vi "AB_Engine_RTDEP_ProjURL_To_NetworkURL.vi"(8 "error in (no error)":errorcluster, 10 "libray ref":refnum<vi>, 11 "Project Refnum":refnum<vi>) -> (0 "error out":errorcluster)   [LabVIEW 2020]
uses:
  <vilib>/variable/NI_Variable.lvlib
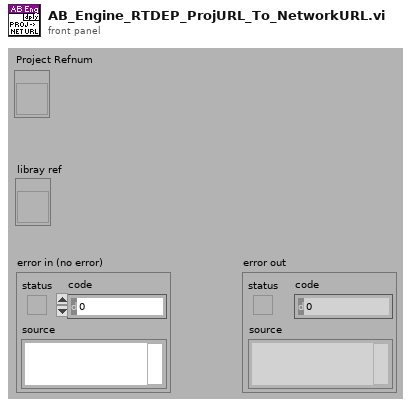
[diagram p1: front panel]
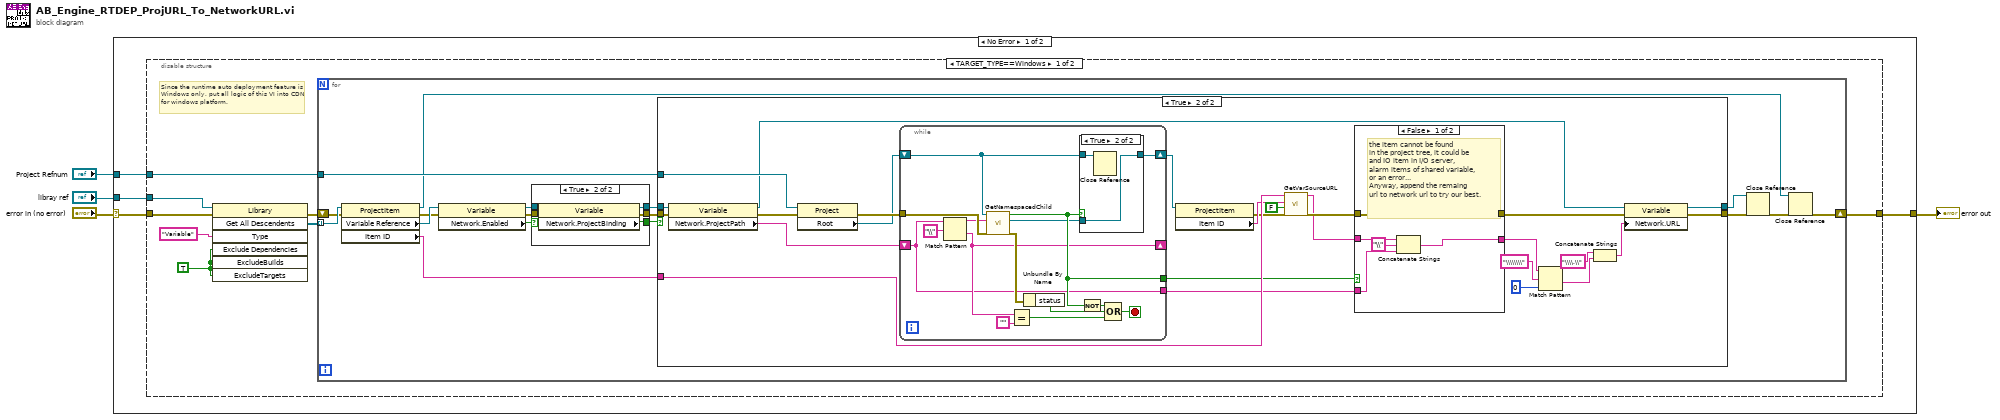
[diagram p0: block diagram]
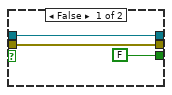
[diagram p2: hidden frame]
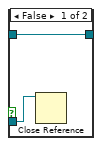
[diagram p5: hidden frame]
diagram:
  n1 = case shown="No Error" "error in (no error)" {
    selector: "error in (no error)" -> [w5 w97]
    tunnel: "Project Refnum" -> [w8 _]
    tunnel: [w7 w97] -> w3
    tunnel: "libray ref" -> [w6 _]
    frame No Error {
      n2 = disable-structure shown="TARGET_TYPE==Windows" {
        disable-tunnel: w8 -> [w16 _]
        disable-tunnel: [w11 w96] -> w7
        disable-tunnel: w6 -> [w10 _]
        disable-tunnel: w5 -> [w9 w96]
        frame condition #0 (active) {
          w14 = TRUE
          # "Since the runtime auto deployment feature is Windows only, put all logic of this VI into CDN for windows platform."
          n3 = invoke class="Library" method="Get All Descendents"(reference=w10, error in=w9, "Type"="Variable", "Exclude Dependencies"=w14, "ExcludeBuilds"=w14, "ExcludeTargets"=w14) -> (error out=w12:errorcluster, "All Descendents"=w13:refnum<vi>[])  [unwired: 1 in, 5 out]
          n4 = for {
            tunnel: w13 -> [w29] mode=indexing
            tunnel: w16 -> [w31]
            shift-right: [w18] -> w11
            shift-left: w12 -> [w26]
            n5 = property class="ProjectItem"(reference=w29, error in=w26) -> (reference out=w27:refnum<vi>, error out=w22:errorcluster, "Variable Reference"=w23:refnum<vi>, "Item ID"=w17:string)
            n6 = property class="Variable"(reference=w23, error in=w22) -> (reference out=w20:refnum<vi>, error out=w21:errorcluster, "Network.Enabled"=w19:bool)
            n7 = case shown="True" w19 {
              tunnel: [FALSE ("Network.ProjectBinding") w41] -> w33
              tunnel: [w36 w40] -> w32
              tunnel: [w34 w39] -> w25
              tunnel: w21 -> [w34 w38]
              tunnel: w20 -> [w36 w37]
              frame False {
              }
              frame True {
                n8 = property class="Variable"(reference=w37, error in=w38) -> (reference out=w40:refnum<vi>, error out=w39:errorcluster, "Network.ProjectBinding"=w41:bool)
              }
            }
            n9 = case shown="True" w33 {
              tunnel: w32 -> [w43 w69]
              tunnel: w31 -> [_ w65]
              tunnel: [w43 w62] -> w30
              tunnel: w25 -> [w42 w67]
              tunnel: [w42 w64] -> w24
              tunnel: w17 -> [_ w61]
              frame False {
              }
              frame True {
                n10 = property class="Variable"(reference=w69, error in=w67) -> (reference out=w63:refnum<vi>, error out=w66:errorcluster, "Network.ProjectPath"=w68:string)
                n11 = property class="Project"(reference=w65, error in=w66) -> (error out=w60:errorcluster, "Root"=w59:refnum<vi>)  [unwired: 1 out]
                n12 = while {
                  shift-right: [w90] -> w49
                  shift-left: w59 -> [w89]
                  shift-right: [w80] -> _
                  shift-left: w68 -> [w78]
                  tunnel: w60 -> [w84]
                  tunnel: [w81] -> w51
                  tunnel: [w78] -> w50
                  stop <- w87 stop-if-true
                  n13 = Match Pattern(string=w78, regular expression="\\") -> (before substring=w79:string, after substring=w80:string)  [unwired: 1 in, 2 out]
                  n14 = call <vilib>:"GetNamespacedChild.vi"("error in"=w84, "name"=w79, "ProjectItem"=w89) -> ("error out"=w83:errorcluster, "child ref"=w77:refnum<vi>, "Found?"=w81:bool)  [unwired: 6 in]
                  n15 = Equal?(x=w80, y="") -> (x = y?=w88:bool)
                  n16 = Unbundle By Name(w83) -> ("status"=w82:bool)
                  n17 = case shown="True" w81 {
                    tunnel: w77 -> [w92 w95]
                    tunnel: [w93 w95] -> w90
                    tunnel: w89 -> [w93 w94]
                    frame False {
                      n18 = Close Reference(reference=w92) -> ()  [unwired: 1 in, 1 out]
                    }
                    frame True {
                      n19 = Close Reference(reference=w94) -> ()  [unwired: 1 in, 1 out]
                    }
                  }
                  n20 = Not(x=w81) -> (.not. x?=w85:bool)
                  n21 = Compound Arithmetic op=OR(w85, w82, w88) -> (w87:bool)
                }
                n22 = property class="ProjectItem"(reference=w49) -> (error out=w47:errorcluster, "Item ID"=w48:string)  [unwired: 1 in, 1 out]
                n23 = call <vilib>:"GetVarSourceURL.vi"("error in"=w47, "targetRelative?"=FALSE, "SourceItemID"=w48, "ItemID"=w61) -> ("error out"=w45:errorcluster, "NetwrokURL"=w44:string)  [unwired: 6 in]
                n24 = case shown="False" w51 {
                  tunnel: [w74 w76] -> w54
                  tunnel: [w71 w75] -> w53
                  tunnel: w50 -> [w73 _]
                  tunnel: w44 -> [w72 w76]
                  tunnel: w45 -> [w71 w75]
                  frame False {
                    # "the item cannot be found \nin the project tree, it could be \nand IO item in I/O server, \nalarm items of shared variable, \nor an error... \nAnyway, append the remaing \nurl to network url to try our best."
                    n25 = Concatenate Strings(w72, "\\" ("string"), w73) -> (w74:string)
                  }
                  frame True {
                  }
                }
                n26 = Match Pattern(string=w54, regular expression="\\\\\\\\" ("string"), offset (0)=0) -> (after substring=w56:string)  [unwired: 3 out]
                n27 = Concatenate Strings("\\\\.\\" ("string"), w56) -> (w52:string)
                n28 = property class="Variable"(reference=w63, error in=w53, "Network.URL"=w52) -> (reference out=w62:refnum<vi>, error out=w64:errorcluster)
              }
            }
            n29 = Close Reference(reference=w30, error in (no error)=w24) -> (error out=w28:errorcluster)
            n30 = Close Reference(reference=w27, error in (no error)=w28) -> (error out=w18:errorcluster)
          }
        }
        frame condition #1 {
        }
      }
    }
    frame Error {
    }
  }
  "error out" <- w3
